vi "New Session Prompt.vi"(10 "Array of channels in":bool[](array[boolean]), 11 "Generic Data Logger.lvlib:Fluke 2625A (Hydra II).lvlib:Fluke 2625A (Hydra II).lvclass":refnum<class "Fluke 2625A (Hydra II).lvclass">) -> (0 "Array of channels out":bool[](array[boolean]), 1 "Time Cluster":cluster{"Warm-Up":dbl, "Measure":dbl}, 3 "Generic Instrument out":refnum<class "Fluke 2625A (Hydra II).lvclass">)   [LabVIEW 2013, in "Generic Data Logger.lvlib" / "Fluke 2625A (Hydra II).lvlib" / "Fluke 2625A (Hydra II).lvclass"]
uses:
  Fluke 2625A (Hydra II).lvclass
  Unit Measurement.ctl
  <instrlib>/Fluke 2625A/Fluke 2625A.lvlib
panel:
  in  "Measure":dbl format="%<%H:%M:%S>t"
  in  "Warm-Up":dbl format="%<%H:%M:%S>t"
  in  "error in (no error)":errorcluster
  in  "Temp Scale":u16(ring)=1 items=["C", "F"]
  out "error out":errorcluster
  in  "Stop Button":bool
  in  "Channel Setup":T1={"Function (5: Temp)"=0, "Channel"=1, "Thermocouple Type (0: J) 2"=0, "Name"=""} {"Thermocouple Type (0: J) 2" items=["J", "K", "E", "T", "N", "R", "S", "B", "C"]; "Channel" min=0 max=20 step=1; "Function (5: Temp)" items=["OFF", "VDC", "VAC", "OHMS", "FREQ", "TEMP"]}
  in  "Array":T1[](array[typedef]) {"Thermocouple Type (0: J) 2" items=["J", "K", "E", "T", "N", "R", "S", "B", "C"]; "Channel" min=0 max=20 step=1; "Function (5: Temp)" items=["OFF", "VDC", "VAC", "OHMS", "FREQ", "TEMP"]}
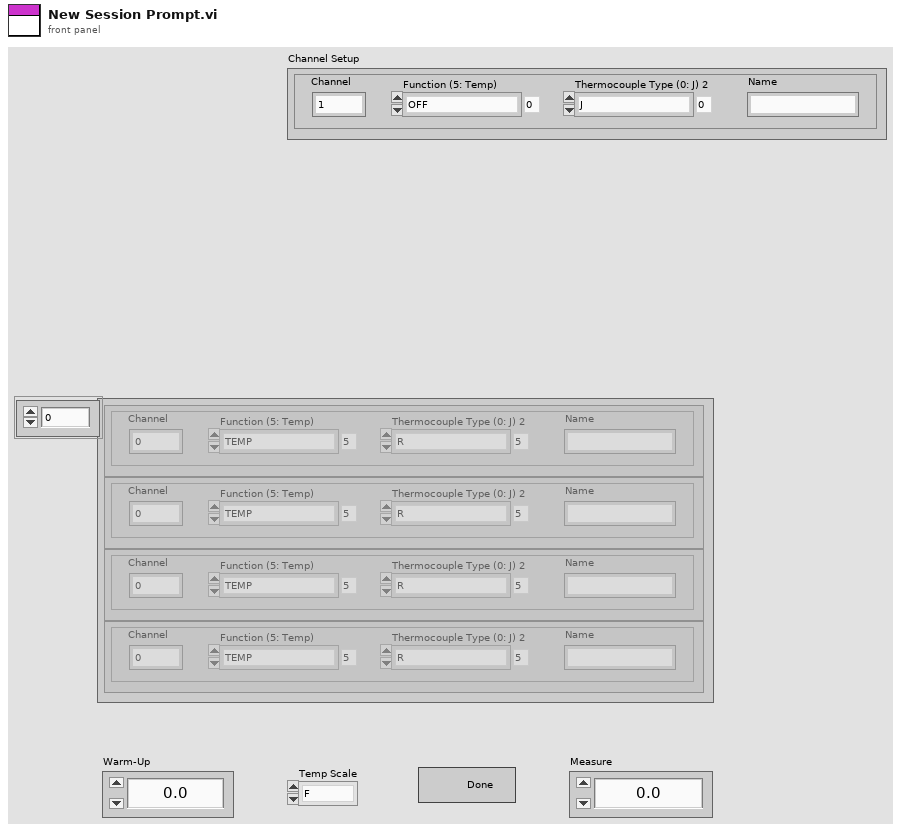
[diagram p1: front panel]
types:
  T1 = typedef "Generic Data Logger.lvlib/Fluke 2625A (Hydra II).lvlib/Fluke 2625A (Hydra II).lvclass/Unit Measurement.ctl" = cluster{"Function (5: Temp)":u16, "Channel":i8, "Thermocouple Type (0: J) 2":u16, "Name":string}
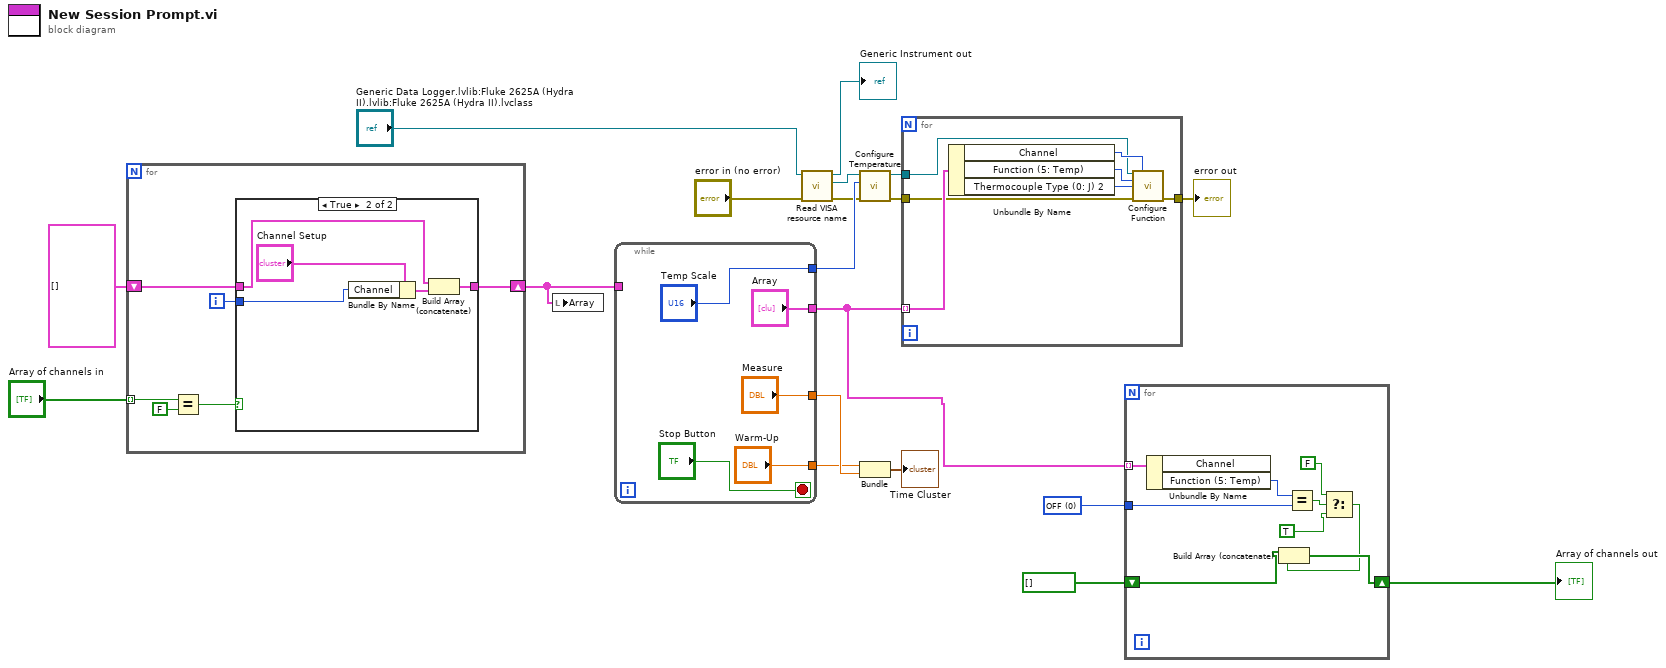
[diagram p0: block diagram]
diagram:
  w2 = u16 0 items=["OFF", "TEMP"] ("Function (5: Temp)")
  n1 = for {
    tunnel: "Array of channels in" -> [w25] mode=indexing
    shift-right: [w22] -> w9
    shift-left: T1[] [] ("Array 3") -> [w23]
    i -> [w20]
    n2 = Equal?(x=w25, y=FALSE) -> (x = y?=w21:bool)
    n3 = case shown="True" w21 {
      tunnel: w23 -> [w26 w31]
      tunnel: [w26 w30] -> w22
      tunnel: w20 -> [_ w28]
      frame False {
      }
      frame True {
        n4 = Bundle By Name(cluster="Channel Setup", "Channel"=w28) -> (w27:T1)
        n5 = Build Array (concatenate)(w31, w27) -> (w30:T1[])
      }
    }
  }
  n6 = local write "Array"(w9) -> ()
  n7 = while {
    tunnel: w9 -> [_]
    tunnel: ["Array"] -> w4
    tunnel: ["Temp Scale"] -> w15
    tunnel: ["Measure"] -> w7
    tunnel: ["Warm-Up"] -> w6
    stop <- "Stop Button" stop-if-true
  }
  n8 = call-dynamic "Read VISA resource name.vi"("error in (no error)"="error in (no error)", "Generic Instrument in"="Generic Data Logger.lvlib:Fluke 2625A (Hydra II).lvlib:Fluke 2625A (Hydra II).lvclass") -> ("error out"=w12:errorcluster, "VISA resource name"=w13:refnum<visa-resource-name>, "Generic Instrument out"=→"Generic Instrument out":refnum<class "Fluke 2625A (Hydra II).lvclass">)  [unwired: 7 in]
  n9 = call <instrlib>:"Configure Temperature.vi"("error in (no error)"=w12, "Temp Scale"=w15, "VISA resource name"=w13) -> ("error out"=w17:errorcluster, "VISA resource name out"=w18:refnum<visa-resource-name>)  [unwired: 6 in, 1 out]
  n10 = Bundle("Warm-Up"=w6, "Measure"=w7) -> (→"Time Cluster":cluster{"Warm-Up":dbl, "Measure":dbl})  [unwired: 1 in]
  n11 = for {
    tunnel: w4 -> [w43] mode=indexing
    tunnel: w18 -> [w37]
    tunnel: w17 -> [w39]
    tunnel: [w38] -> w16
    n12 = Unbundle By Name(w43) -> ("Channel"=w40:i8, "Function (5: Temp)"=w42:u16, "Thermocouple Type (0: J) 2"=w41:u16)
    n13 = call <instrlib>:"Configure Function.vi"("VISA resource name"=w37, "Channel"=w40, "Function (5: Temp)"=w42, "Thermocouple Type (0: J) 2"=w41, "error in (no error)"=w39) -> ("error out"=w38:errorcluster)  [unwired: 7 in, 3 out]
  }
  "error out" <- w16
  n14 = for {
    tunnel: w4 -> [w52] mode=indexing
    shift-right: [w48] -> w1
    shift-left: bool[] [] ("Array of channels in") -> [w49]
    tunnel: w2 -> [w50]
    n15 = Unbundle By Name(w52) -> ("Function (5: Temp)"=w51:u16)  [unwired: 1 out]
    n16 = Equal?(x=w51, y=w50) -> (x = y?=w47:bool)
    n17 = Select(t=FALSE, s=w47, f=TRUE) -> (s? t:f=w44:bool)
    n18 = Build Array (concatenate)(w49, w44) -> (w48:bool[])
  }
  "Array of channels out" <- w1
